vi "gm_sqlite_write_time.vi"(8 "error in (no error)":errorcluster, 9 "output cluster timestamp":timestamp, 10 "Database File":string, 11 "Output - Cluster gas":T1 {"GM TS-2[°C]" format="%.2g"; "GM TS-1 [°C]" format="%.2g"; "GM DS-1 [bar]" format="%.4g"; "GM DS-2 [bar]" format="%.4g"; "GA1 h2 [%]" format="%.2g"; "GA1 co2 [%]" format="%.2g"; "GA1 ch4 [%]" format="%.2g"}) -> (0 "error out":errorcluster)   [LabVIEW 2011]
uses:
  Output - Cluster gas.ctl
  gas_values.ctl
panel:
  # "qualitätsmessung"
  # "quantitätsmessung"
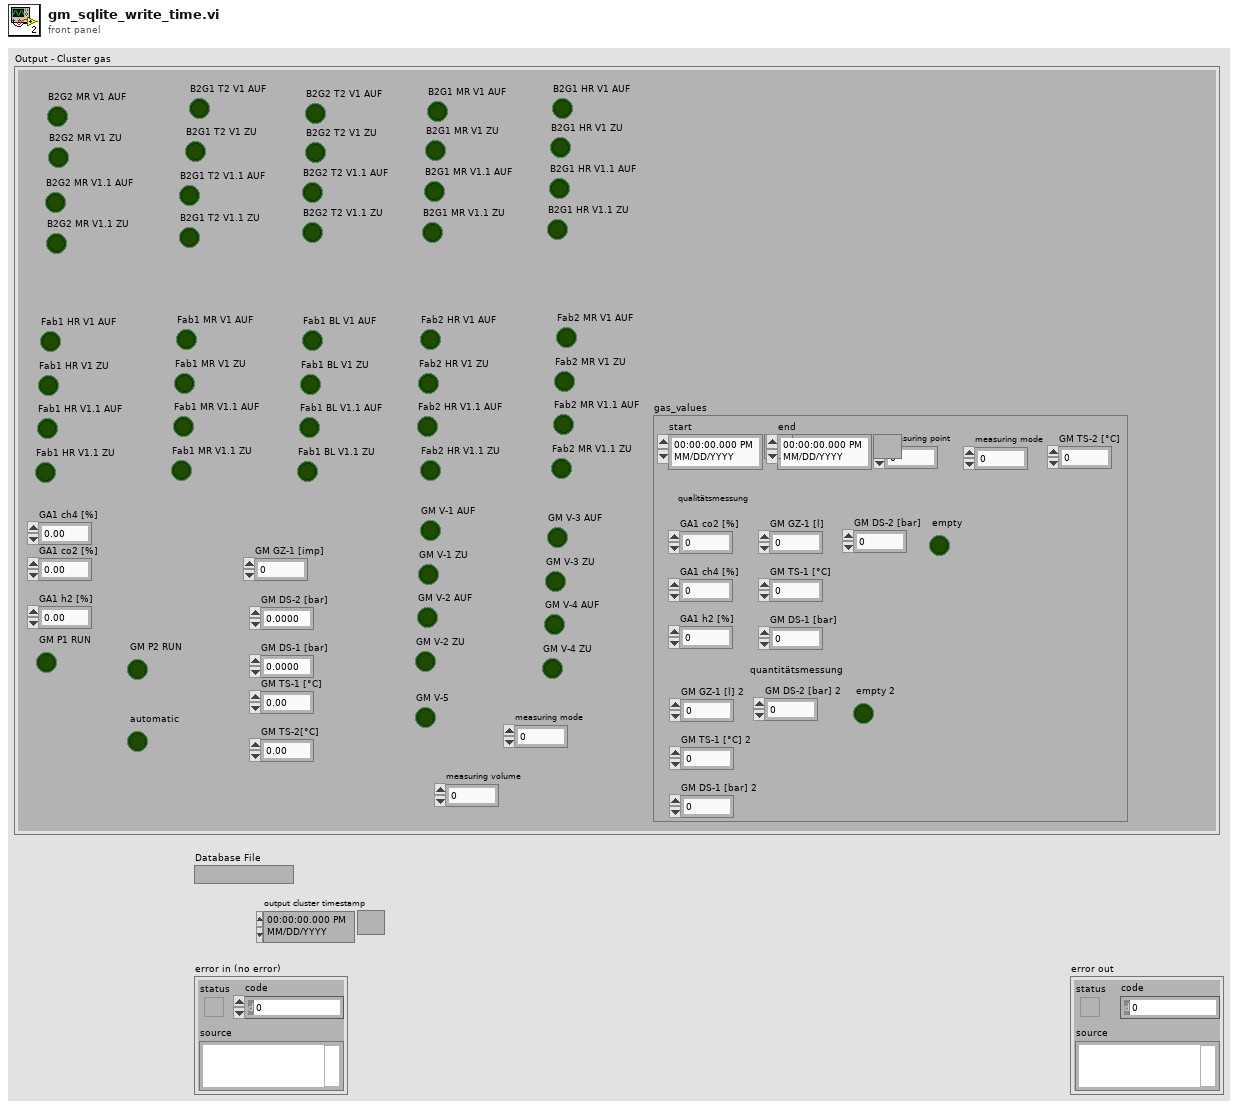
[diagram p1: front panel]
types:
  T1 = typedef "Output - Cluster gas.ctl" = cluster{"B2G2 MR V1.1 AUF":bool, "B2G2 MR V1.1 ZU":bool, "B2G2 MR V1 AUF":bool, "B2G2 MR V1 ZU":bool, "B2G1 T2 V1 AUF":bool, "B2G1 T2 V1 ZU":bool, "B2G1 T2 V1.1 AUF":bool, "B2G1 T2 V1.1 ZU":bool, "B2G2 T2 V1 AUF":bool, "B2G2 T2 V1 ZU":bool, "B2G2 T2 V1.1 ZU":bool, "B2G2 T2 V1.1 AUF":bool, "B2G1 MR V1 AUF":bool, "B2G1 MR V1 ZU":bool, "B2G1 MR V1.1 AUF":bool, "B2G1 MR V1.1 ZU":bool, "B2G1 HR V1 AUF":bool, "B2G1 HR V1 ZU":bool, "B2G1 HR V1.1 AUF":bool, "B2G1 HR V1.1 ZU":bool, "Fab1 HR V1 AUF":bool, "Fab1 HR V1 ZU":bool, "Fab1 HR V1.1 AUF":bool, "Fab1 HR V1.1 ZU":bool, "Fab1 MR V1 AUF":bool, "Fab1 MR V1 ZU":bool, "Fab1 MR V1.1 AUF":bool, "Fab1 MR V1.1 ZU":bool, "Fab1 BL V1 AUF":bool, "Fab1 BL V1 ZU":bool, "Fab1 BL V1.1 AUF":bool, "Fab1 BL V1.1 ZU":bool, "Fab2 HR V1 AUF":bool, "Fab2 HR V1 ZU":bool, "Fab2 HR V1.1 AUF":bool, "Fab2 HR V1.1 ZU":bool, "Fab2 MR V1 AUF":bool, "Fab2 MR V1 ZU":bool, "Fab2 MR V1.1 AUF":bool, "Fab2 MR V1.1 ZU":bool, "GA1 ch4 [%]":dbl, "GA1 co2 [%]":dbl, "GA1 h2 [%]":dbl, "GM P1 RUN":bool, "GM V-1 AUF":bool, "GM V-1 ZU":bool, "GM V-2 AUF":bool, "GM V-2 ZU":bool, "GM V-3 AUF":bool, "GM V-3 ZU":bool, "GM V-4 AUF":bool, "GM V-4 ZU":bool, "GM P2 RUN":bool, "GM GZ-1 [imp]":u32, "GM DS-2 [bar]":dbl, "GM DS-1 [bar]":dbl, "GM TS-1 [°C]":dbl, "GM TS-2[°C]":dbl, "gas_values":T2, "measuring mode":u8, "GM V-5":bool, "measuring volume":dbl, "automatic":bool}
  T2 = typedef "gas_values.ctl" = cluster{"start":timestamp, "GM DS-2 [bar]":dbl, "GA1 ch4 [%]":dbl, "GA1 co2 [%]":dbl, "GA1 h2 [%]":dbl, "GM DS-1 [bar]":dbl, "GM TS-1 [°C]":dbl, "GM TS-2 [°C]":dbl, "GM GZ-1 [l]":dbl, "measuring point":u8, "end":timestamp, "empty":bool, "GM GZ-1 [l] 2":dbl, "GM TS-1 [°C] 2":dbl, "GM DS-1 [bar] 2":dbl, "GM DS-2 [bar] 2":dbl, "empty 2":bool, "measuring mode":u8}
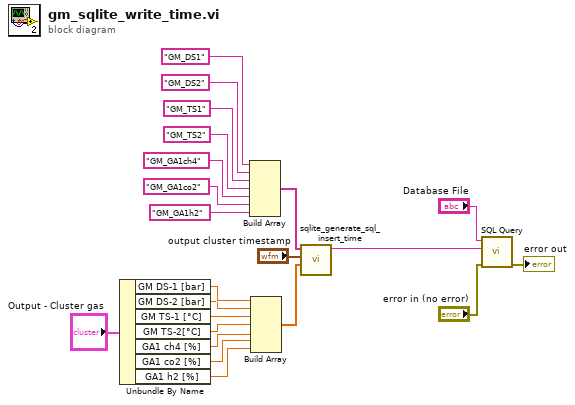
[diagram p0: block diagram]
diagram:
  n1 = Unbundle By Name("Output - Cluster gas") -> ("GM DS-1 [bar]"=w21:dbl, "GM DS-2 [bar]"=w20:dbl, "GM TS-1 [°C]"=w19:dbl, "GM TS-2[°C]"=w18:dbl, "GA1 ch4 [%]"=w17:dbl, "GA1 co2 [%]"=w16:dbl, "GA1 h2 [%]"=w15:dbl)
  n2 = Build Array("GM_DS1" ("SQL Query"), "GM_DS2" ("SQL Query"), "GM_TS1" ("SQL Query"), "GM_TS2" ("SQL Query"), "GM_GA1ch4" ("SQL Query"), "GM_GA1co2" ("SQL Query"), "GM_GA1h2" ("SQL Query")) -> (w4:string[])
  n3 = Build Array(w21, w20, w19, w18, w17, w16, w15) -> (w2:dbl[])
  n4 = call "sqlite_generate_sql_insert_time.vi"("Array"=w2, "output cluster timestamp"="output cluster timestamp", "Array 2"=w4) -> ("String"=w1:string)  [unwired: 8 in]
  n5 = call "SQL Query.vi"("error in (no error)"="error in (no error)", "SQL Query"=w1, "Database File"="Database File") -> ("error out"=→"error out":errorcluster)  [unwired: 6 in, 2 out]
